vi "BinaryStrings.vi"(6 "Array":T1(array[cluster])=[{"Numeric"=1.0, "String"="ß\u0000Ã¶\u0000\u0001\u0000\u0000±®¥", "Smith Plot"=bytes[4630]}], 8 "Array Of Plots":picture[](array[picture])=[bytes[4630], bytes[746]], 9 "Cluster":T2={"Numeric"=112233.0, "String"="姓葸\u0000枚\u0000\u0001\u0000\u0000碑ぅ", "Smith Plot"=bytes[4630]}, 10 "String 2":string="Ë\u0000«ì²\u0000’†\u0000‰Œ¼½¾", 11 "String":string="\u0001\u0000œ£§\u0004\u0010\u0012\u0000\u0016\u0019\u0018\u0000\u001a\u001dÆ§§") -> (3 "Got Expected Default Values":bool)   [LabVIEW 2009]
panel:
  in  "stop":bool
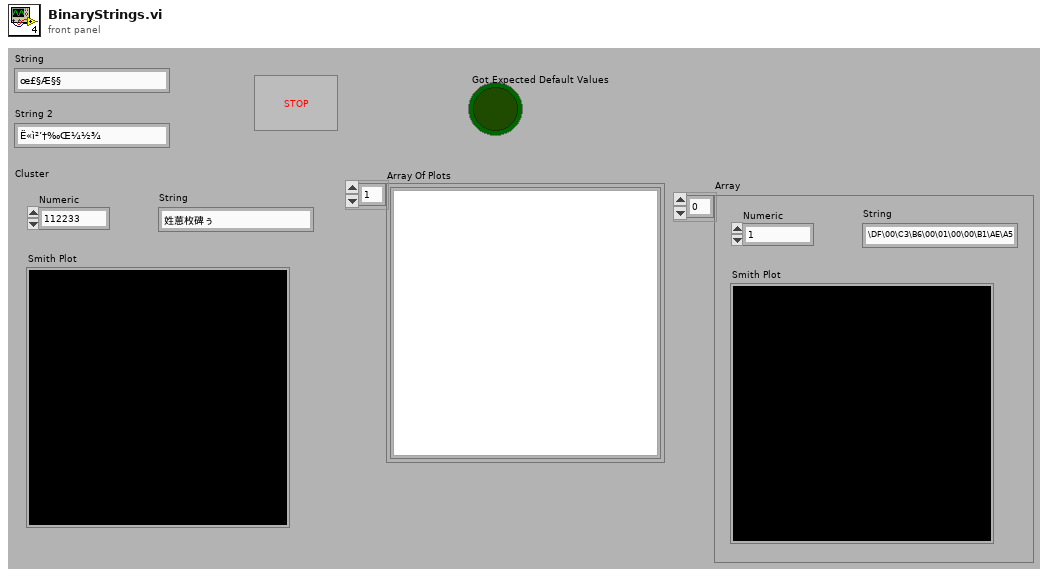
[diagram p1: front panel]
types:
  T1 = cluster{"Numeric":dbl, "String":string, "Smith Plot":picture}[]
  T2 = cluster{"Numeric":dbl, "String":string, "Smith Plot":picture}
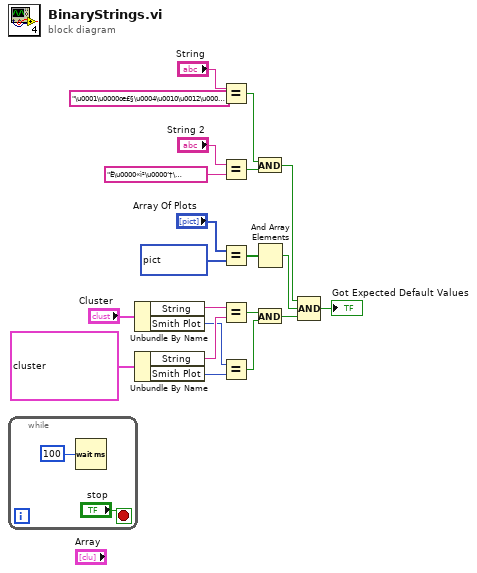
[diagram p0: block diagram]
diagram:
  n1 = while {
    stop <- "stop" stop-if-true
    n2 = Wait (ms)(milliseconds to wait=u32 100) -> ()  [unwired: 1 out]
  }
  n3 = Unbundle By Name("Cluster") -> ("String"=w7:string, "Smith Plot"=w5:picture)
  n4 = Unbundle By Name(T2 {"Numeric"=112233.0, "String"="姓葸\u0000枚\u0000\u0001\u0000\u0000碑ぅ", "Smith Plot"=bytes[4630]} ("Cluster")) -> ("String"=w6:string, "Smith Plot"=w4:picture)
  n5 = Equal?(x="String", y="\u0001\u0000œ£§\u0004\u0010\u0012\u0000\u0016\u0019\u0018\u0000\u001a\u001dÆ§§" ("String")) -> (x = y?=w17:bool)
  n6 = Equal?(x="String 2", y="Ë\u0000«ì²\u0000’†\u0000‰Œ¼½¾" ("String 2")) -> (x = y?=w16:bool)
  n7 = Equal?(x="Array Of Plots", y=picture[] [bytes[4630], bytes[3948], bytes[1226], bytes[4718], bytes[746]] ("Array Of Plots")) -> (x = y?=w13:bool[])
  n8 = Equal?(x=w7, y=w6) -> (x = y?=w3:bool)
  n9 = Equal?(x=w5, y=w4) -> (x = y?=w2:bool)
  n10 = And(x=w17, y=w16) -> (x .and. y?=w12:bool)
  n11 = And Array Elements(Boolean array=w13) -> (logical AND=w11:bool)
  n12 = And(x=w3, y=w2) -> (x .and. y?=w1:bool)
  n13 = Compound Arithmetic op=AND(w12, w11, w1) -> (→"Got Expected Default Values":bool)
